vi "Untitled 5 (SubVI).vi"(9 "in":bool, 10 "?":bool, 11 "X":i32) -> (2 "Boolean":bool, 3 "out":string)   [LabVIEW 2020]
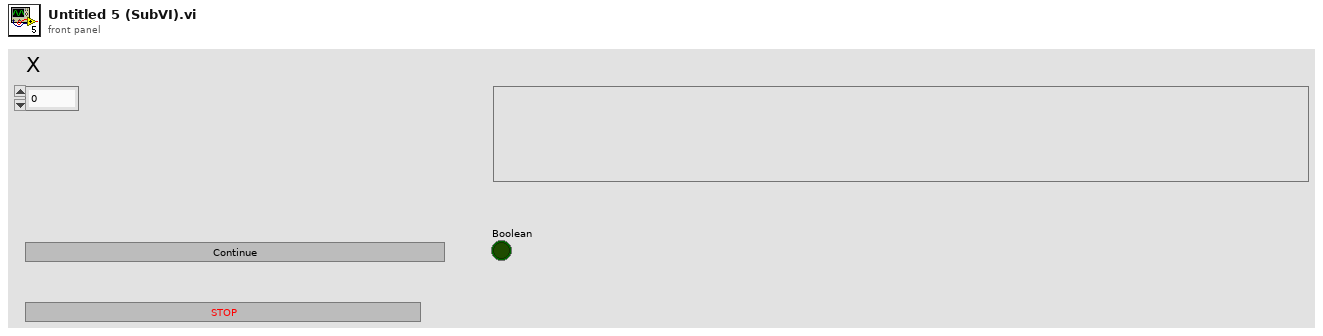
[diagram p1: front panel]
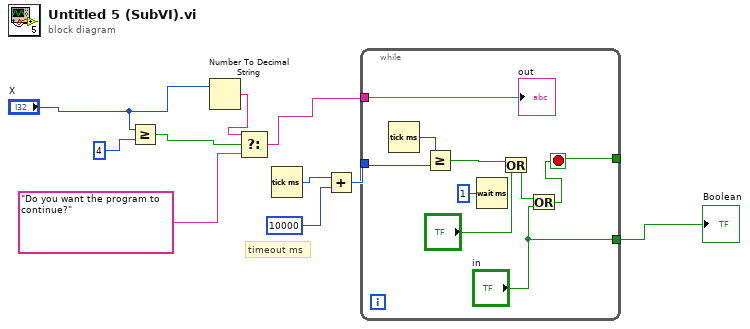
[diagram p0: block diagram]
diagram:
  # "timeout ms"
  n1 = Greater Or Equal?(x="X", y=4) -> (x >= y?=w7:bool)
  n2 = Number To Decimal String(number="X") -> (decimal integer string=w6:string)  [unwired: 1 in]
  n3 = Select(t=w6, s=w7, f="Do you want the program to continue?") -> (s? t:f=w5:string)
  n4 = Tick Count (ms)() -> (millisecond timer value=w3:u32)
  n5 = Add(x=w3, y=u32 10000) -> (x+y=w2:u32)
  n6 = while {
    tunnel: w2 -> [w18]
    tunnel: [w12] -> _
    tunnel: w5 -> [w14]
    tunnel: ["in"] -> w10
    stop <- w12 stop-if-true
    n7 = Tick Count (ms)() -> (millisecond timer value=w17:u32)
    n8 = Greater Or Equal?(x=w17, y=w18) -> (x >= y?=w16:bool)
    n9 = Wait (ms)(milliseconds to wait=u32 1 ("millisecond timer value")) -> ()  [unwired: 1 out]
    n10 = Or(x=w16, y="?") -> (x .or. y?=w13:bool)
    n11 = Or(x=w13, y="in") -> (x .or. y?=w12:bool)
    "out" <- w14
  }
  "Boolean" <- w10
